vi "gopro test.vi"() -> ()   [LabVIEW 2015]
uses:
  GoPro Status.ctl
  GoPro Mode.ctl
  GoPro FPS.ctl
  GoPro Resolution.ctl
  GoPro Video FOV.ctl
  GoPro Photo Resolution.ctl
panel:
  in  "PV?":bool
  out "GoPro Status":T1={"State"=enum."Menu", "Record Elapsed"="", "Record Remaining"=0, "On?"=FALSE, "sx"="", "cc"="", "cv"="", "se"="", "Recording?"=FALSE, "Video Files"=0, "Pics Remaining"=0, "Pic Files"=0, "FPS"=enum."120 FPS", "Resolution"=enum."1080p", "Spot Metering?"=FALSE, "Vid FOV"=enum."Wide", "Photo Resolution"=enum."10 MP W", "Beep Vol"=enum."OFF"}
  out "sx byte array":u8[](array[numeric])
  out "length":i32
  out "Numeric":i32
  out "sx":string
  out "cc":string
  out "cv":string
  out "se":string
  in  "stop":bool
  in  "On?":bool
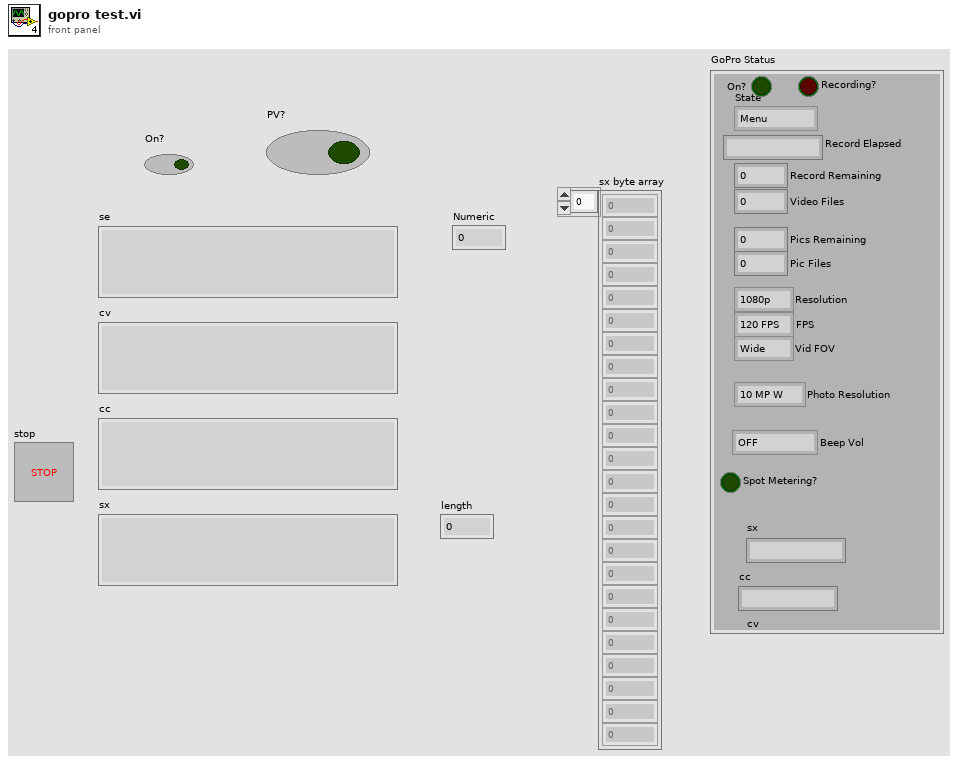
[diagram p1: front panel]
types:
  T1 = typedef "GoPro Status.ctl" = cluster{"State":T2, "Record Elapsed":string, "Record Remaining":i32, "On?":bool, "sx":string, "cc":string, "cv":string, "se":string, "Recording?":bool, "Video Files":i32, "Pics Remaining":i32, "Pic Files":i32, "FPS":T3, "Resolution":T4, "Spot Metering?":bool, "Vid FOV":T5, "Photo Resolution":T6, "Beep Vol":enum16{"OFF", "70%", "100%", "UNKOWN"}}
  T2 = typedef "GoPro Mode.ctl" = enum16{"UNKNOWN", "Video", "Photo", "Time Lapse", "Timer Delay", "Menu"}
  T3 = typedef "GoPro FPS.ctl" = enum16{"120 FPS", "60 FPS", "30 FPS", "UNKNOWN"}
  T4 = typedef "GoPro Resolution.ctl" = enum16{"1080p", "960p", "720p", "WVGA", "UNKNOWN"}
  T5 = typedef "GoPro Video FOV.ctl" = enum16{"Wide", "Medium", "Narrow", "UNKNOWN"}
  T6 = typedef "GoPro Photo Resolution.ctl" = enum16{"10 MP W", "7 MP W", "5 MP M", "UNKNOWN"}
  T7 = typedef "GoPro DevRef.ctl" = cluster{"name":string, "pw":string, "client handle":T8}
  T8 = typedef "LabVIEWHTTPClient.lvlib/ClientHandle.ctl" = refnum<k1>
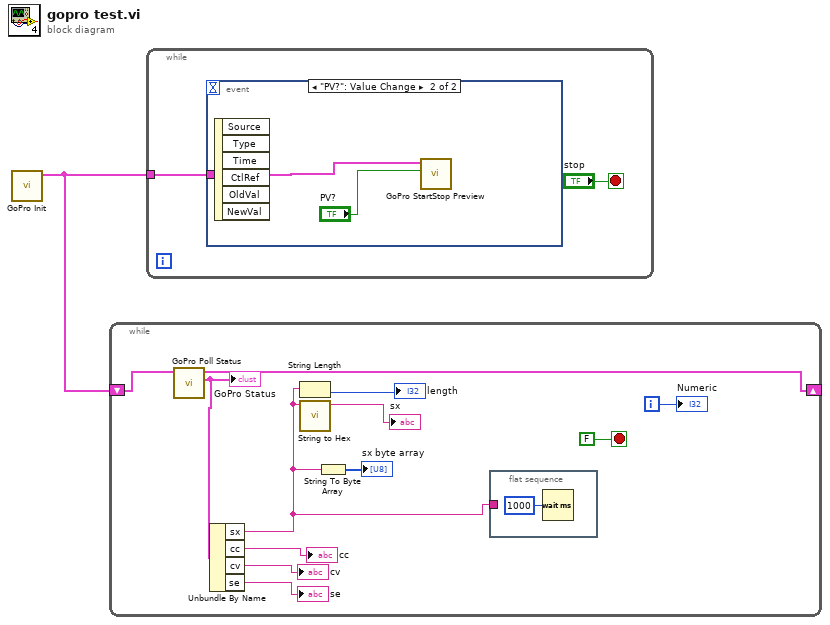
[diagram p0: block diagram]
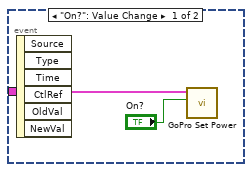
[diagram p2: hidden frame]
diagram:
  n1 = call "GoPro Init.vi"() -> ("Gopro DevRef"=w1:T7)  [unwired: 10 in, 1 out]
  n2 = while {
    shift-right: [w12] -> _
    shift-left: w1 -> [w11]
    i -> [w10]
    stop <- FALSE stop-if-true
    n3 = call "GoPro Poll Status.vi"("Gopro DevRef"=w11) -> ("GoPro Status"=w7:T1, "Output DevRef"=w12:T7)  [unwired: 8 in, 1 out]
    "GoPro Status" <- w7
    n4 = Unbundle By Name(w7) -> ("sx"=w2:string, "cc"=→"cc":string, "cv"=→"cv":string, "se"=→"se":string)
    n5 = String Length(string=w2) -> (length=→"length":i32)
    n6 = call "String to Hex.vi"("body"=w2) -> ("hex string"=→"sx":string)  [unwired: 10 in]
    n7 = String To Byte Array(string=w2) -> (unsigned byte array=→"sx byte array":u8[])
    n8 = flat-sequence {
      tunnel: w2 -> [_]
      frame #0 {
        n9 = Wait (ms)(milliseconds to wait=u32 1000) -> ()  [unwired: 1 out]
      }
    }
    "Numeric" <- w10
  }
  n10 = while {
    tunnel: w1 -> [w16]
    stop <- "stop" stop-if-true
    n11 = event shown="[1] \"PV?\": Value Change" {
      selector: _ -> [_ _]
      dyn-events: _ -> [_ _]
      timeout: _ -> [_ _]
      tunnel: w16 -> [w18 w20]
      event "On?": Value Change {
        n12 = event-data() -> ()  [unwired: 1 in, 6 out]
        n13 = call "GoPro Set Power.vi"("On?"="On?", "Gopro DevRef"=w18) -> ()  [unwired: 9 in, 1 out]
      }
      event "PV?": Value Change {
        n14 = event-data() -> ()  [unwired: 1 in, 6 out]
        n15 = call "GoPro StartStop Preview.vi"("PV?"="PV?", "Gopro DevRef"=w20) -> ()  [unwired: 9 in, 1 out]
      }
    }
  }
